vi "swap tracking spot.vi"(0 "N spot tracker in":T5, 1 "tracking?":bool=TRUE, 2 "current location":T2, 5 "tracking state in":T6={"x state"={"pos estimate"=0.0, "v estimate"=0.0, "weighted position error sum"=0.0, "photon count"=0, "transmit tick count"=0, "axis number"=0, "px (levels^2)"=0.0, "pxv (levels^2/ticks)"=0.0, "pv (levels^2/ticks^2)"=0.0, "vel diff (levels^2/ticks^3)"=0.0, "gx"=0.0, "rtwiddle"=0.0, "photon count ch0"=0, "photon count ch1"=0, "Dx - for pos only k-f"=0.0}, "y state"={"pos estimate"=0.0, "v estimate"=0.0, "weighted position error sum"=0.0, "photon count"=0, "transmit tick count"=0, "axis number"=1, "px (levels^2)"=0.0, "pxv (levels^2/ticks)"=0.0, "pv (levels^2/ticks^2)"=0.0, "vel diff (levels^2/ticks^3)"=0.0, "gx"=0.0, "rtwiddle"=0.0, "photon count ch0"=0, "photon count ch1"=0, "Dx - for pos only k-f"=0.0}, "z state"={"pos estimate"=0.0, "v estimate"=0.0, "weighted position error sum"=0.0, "photon count"=0, "transmit tick count"=0, "axis number"=2, "px (levels^2)"=0.0, "pxv (levels^2/ticks)"=0.0, "pv (levels^2/ticks^2)"=0.0, "vel diff (levels^2/ticks^3)"=0.0, "gx"=0.0, "rtwiddle"=0.0, "photon count ch0"=0, "photon count ch1"=0, "Dx - for pos only k-f"=0.0}, "spot number"=0}, 7 "reset flags":u8, 9 "new circle":bool, 11 "permission to swap states":bool, 12 "spot location constraints":T3=[{"spot number"=0, "active"=FALSE, "x max"=0, "x min"=0, "y max"=0, "y min"=0}, {"spot number"=0, "active"=FALSE, "x max"=0, "x min"=0, "y max"=0, "y min"=0}, {"spot number"=0, "active"=FALSE, "x max"=0, "x min"=0, "y max"=0, "y min"=0}, {"spot number"=0, "active"=FALSE, "x max"=0, "x min"=0, "y max"=0, "y min"=0}], 13 "update tracking? in":T1) -> (3 "update tracking? out":T1, 4 "N spot tracker out":T5, 6 "tracking state out":T6={"x state"={"pos estimate"=0.0, "v estimate"=0.0, "weighted position error sum"=0.0, "photon count"=0, "transmit tick count"=0, "axis number"=0, "px (levels^2)"=0.0, "pxv (levels^2/ticks)"=0.0, "pv (levels^2/ticks^2)"=0.0, "vel diff (levels^2/ticks^3)"=0.0, "gx"=0.0, "rtwiddle"=0.0, "photon count ch0"=0, "photon count ch1"=0, "Dx - for pos only k-f"=0.0}, "y state"={"pos estimate"=0.0, "v estimate"=0.0, "weighted position error sum"=0.0, "photon count"=0, "transmit tick count"=0, "axis number"=1, "px (levels^2)"=0.0, "pxv (levels^2/ticks)"=0.0, "pv (levels^2/ticks^2)"=0.0, "vel diff (levels^2/ticks^3)"=0.0, "gx"=0.0, "rtwiddle"=0.0, "photon count ch0"=0, "photon count ch1"=0, "Dx - for pos only k-f"=0.0}, "z state"={"pos estimate"=0.0, "v estimate"=0.0, "weighted position error sum"=0.0, "photon count"=0, "transmit tick count"=0, "axis number"=2, "px (levels^2)"=0.0, "pxv (levels^2/ticks)"=0.0, "pv (levels^2/ticks^2)"=0.0, "vel diff (levels^2/ticks^3)"=0.0, "gx"=0.0, "rtwiddle"=0.0, "photon count ch0"=0, "photon count ch1"=0, "Dx - for pos only k-f"=0.0}, "spot number"=0}, 10 "use photons to track":bool)   [LabVIEW 2010]
uses:
  kalman 3-axis state.ctl
  integrating single axis kalman state.ctl
  kalman N spot state.ctl
  spot location constraints.ctl
  spot location constraint.ctl
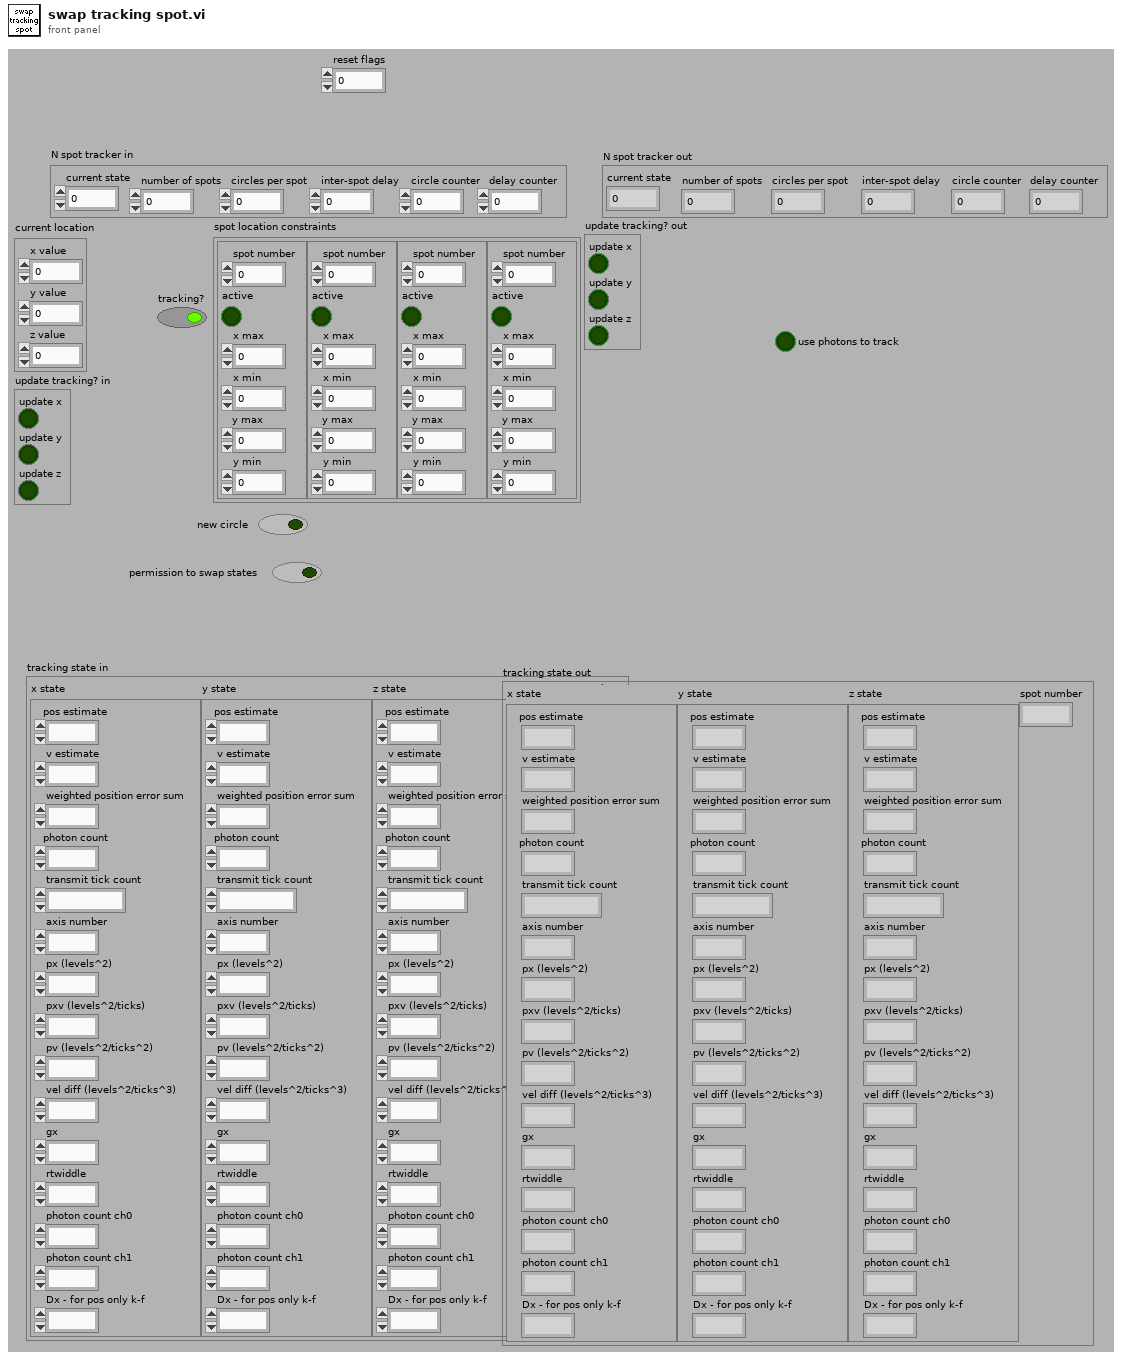
[diagram p1: front panel]
types:
  T1 = cluster{"update x":bool, "update y":bool, "update z":bool}
  T2 = cluster{"x value":i16, "y value":i16, "z value":i16}
  T3 = typedef "spot location constraints.ctl" = T4[]
  T4 = typedef "spot location constraint.ctl" = cluster{"spot number":i8, "active":bool, "x max":i16, "x min":i16, "y max":i16, "y min":i16}
  T5 = typedef "kalman N spot state.ctl" = cluster{"current state":u8, "number of spots":u8, "circles per spot":u16, "inter-spot delay":u8, "circle counter":u16, "delay counter":u8}
  T6 = typedef "kalman 3-axis state.ctl" = cluster{"x state":T7, "y state":T7, "z state":T7, "spot number":u8}
  T7 = typedef "integrating single axis kalman state.ctl" = cluster{"pos estimate":fxp<+/-,32,16>, "v estimate":fxp<+/-,16,0>, "weighted position error sum":fxp<+/-,32,32>, "photon count":u32, "transmit tick count":u32, "axis number":u8, "px (levels^2)":fxp<+,32,19>, "pxv (levels^2/ticks)":fxp<+,32,2>, "pv (levels^2/ticks^2)":fxp<+,32,-14>, "vel diff (levels^2/ticks^3)":fxp<+,24,-22>, "gx":fxp<+,16,8>, "rtwiddle":fxp<+,16,26>, "photon count ch0":u32, "photon count ch1":u32, "Dx - for pos only k-f":fxp<+,32,19>}
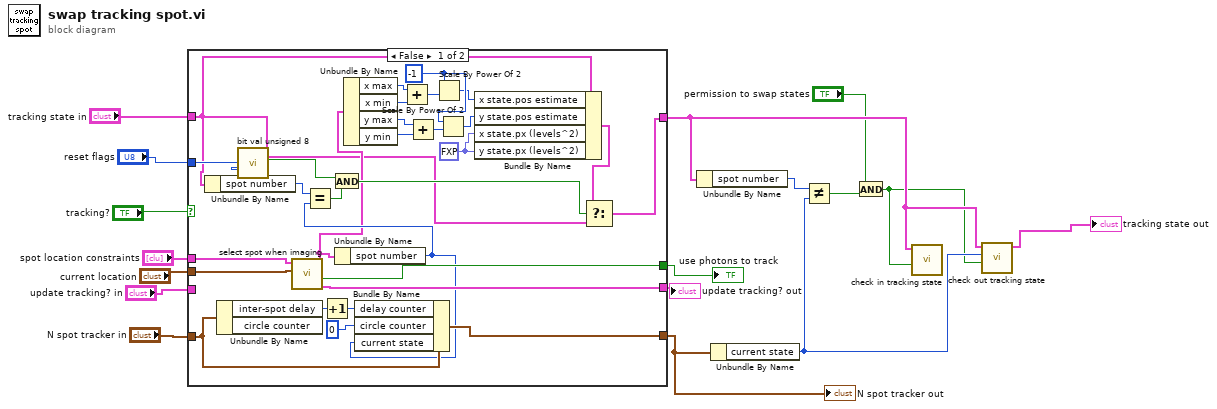
[diagram p0: block diagram]
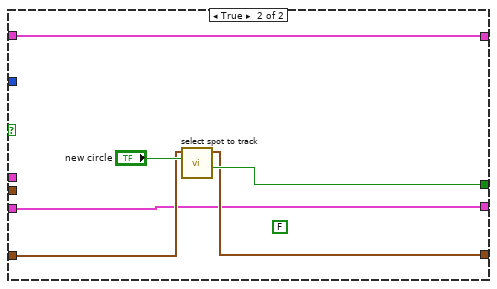
[diagram p2: hidden frame]
diagram:
  n1 = case shown="False" "tracking?" {
    tunnel: [w39 w51] -> w15
    tunnel: [w42 w50] -> w14
    tunnel: "N spot tracker in" -> [w43 w49]
    tunnel: "spot location constraints" -> [w41 _]
    tunnel: "current location" -> [w40 _]
    tunnel: [w38 w48] -> w11
    tunnel: "update tracking? in" -> [_ w48]
    tunnel: "tracking state in" -> [w20 w47]
    tunnel: [w18 w47] -> w6
    tunnel: "reset flags" -> [w33 _]
    frame False {
      w19 = fxp<+,32,19> 0.0 ("x state.px (levels^2)")
      w24 = -1 ("n")
      n2 = Unbundle By Name(w20) -> ("spot number"=w34:u8)
      n3 = Unbundle By Name(w43) -> ("inter-spot delay"=w46:u8)  [unwired: 1 out]
      n4 = call "bit val unsigned 8.vi"("bit num"=w34, "x"=w33) -> ("BV"=w35:bool)  [unwired: 9 in]
      n5 = call "select spot when imaging.vi"("current location"=w40, "spot location constraints"=w41) -> ("update tracking?"=w38:T1, "acquire"=w39:bool, "selected spot"=w31:T4)  [unwired: 7 in]
      n6 = Increment(x=w46) -> (x+1=w45:u8)
      n7 = Unbundle By Name(w31) -> ("spot number"=w37:i8)
      n8 = Equal?(x=w34, y=w37) -> (x = y?=w36:bool)
      n9 = And(x=w35, y=w36) -> (x .and. y?=w32:bool)
      n10 = Unbundle By Name(w31) -> ("x max"=w29:i16, "x min"=w30:i16, "y max"=w28:i16, "y min"=w27:i16)
      n11 = Bundle By Name(cluster=w43, "delay counter"=w45, "circle counter"=u8 0, "current state"=w37) -> (w42:T5)
      n12 = Add(x=w29, y=w30) -> (x+y=w26:i16)
      n13 = Add(x=w28, y=w27) -> (x+y=w25:i16)
      n14 = Scale By Power Of 2(n=w24, x=w26) -> (x*2^n=w23:i16)
      n15 = Scale By Power Of 2(n=w24, x=w25) -> (x*2^n=w22:i16)
      n16 = Bundle By Name(cluster=w20, "x state.pos estimate"=w23, "y state.pos estimate"=w22, "x state.px (levels^2)"=w19, "y state.px (levels^2)"=w19) -> (w21:T6)
      n17 = Select(t=w21, s=w32, f=w20) -> (s? t:f=w18:T6)
    }
    frame True {
      (unwired) FALSE ("set state?")
      n18 = call "select spot to track.vi"("new circle"="new circle", "N spot tracker in"=w49) -> ("use photons to track"=w51:bool, "N spot tracker out"=w50:T5)  [unwired: 8 in]
    }
  }
  "use photons to track" <- w15
  "N spot tracker out" <- w14
  "update tracking? out" <- w11
  n19 = Unbundle By Name(w6) -> ("spot number"=w5:u8)
  n20 = Unbundle By Name(w14) -> ("current state"=w4:u8)
  n21 = Not Equal?(x=w5, y=w4) -> (x != y?=w3:bool)
  n22 = And(x="permission to swap states", y=w3) -> (x .and. y?=w1:bool)
  n23 = call "check in tracking state.vi"("check in state"=w1, "state to check in"=w6) -> ()  [unwired: 10 in]
  n24 = call "check out tracking state.vi"("check out state"=w1, "state number"=w4, "previous state"=w6) -> ("state out"=→"tracking state out":T6)  [unwired: 8 in]
